vi "SDO_6041_Lese_Statusword.vi"(8 "error in (no error)":errorcluster, 11 "SDO object in":refnum<k20>) -> (0 "error out":errorcluster, 1 "U16 data":u16, 2 "completion code":u32 format="%.0x", 3 "SDO object out":refnum<k20>)   [LabVIEW 2014]
uses:
  <vilib>/CANopenLib/CANOPEN.llb/CANopen SDO Read [U16].vi
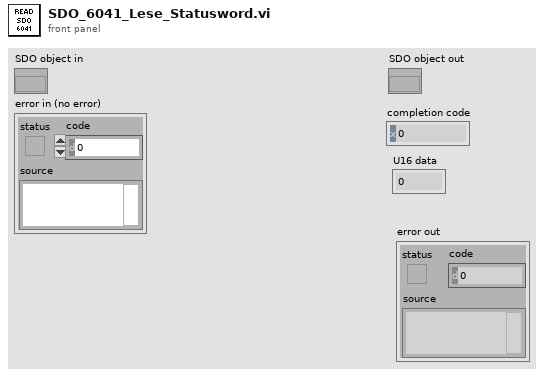
[diagram p1: front panel]
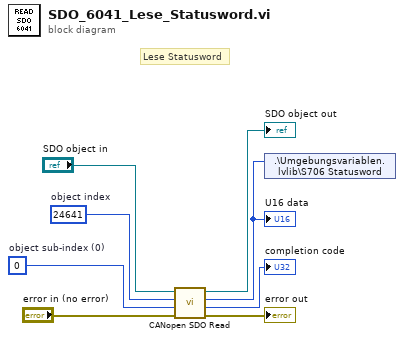
[diagram p0: block diagram]
diagram:
  w6 = u8 0  # object sub-index (0)
  w7 = u16 24641  # object index
  # "Lese Statusword"
  n1 = call-poly <vilib>:"CANopen SDO Read.vi"("error in (no error)"="error in (no error)", "object sub-index (0)"=w6, "object index"=w7, "SDO object in"="SDO object in") -> ("error out"=→"error out":errorcluster, "completion code"=→"completion code":u32, "U16 data"=w1:u16, "SDO object out"=→"SDO object out":refnum<k20>)  [unwired: 4 in]
  "U16 data" <- w1
  n2 = shared-variable ".\\Umgebungsvariablen.lvlib\\S706 Statusword"(w1) -> ()  [unwired: 1 in, 1 out]
